vi "Voltage Update.vi"(7 "shared variable refnum in":refnum<k21>, 8 "error in (no error)":errorcluster, 9 "Amplifier Gain":dbl=1.0 min=-15.0 max=15.0, 10 "Voltage Output":dbl(slide) min=-50.0 max=50.0 scale=-45.0..45.0, 11 "Physical Channel":tag="Dev2/ao0") -> (0 "error out":errorcluster, 2 "DAQ output":dbl(slide)=-0.0 min=-3.5 max=3.5 scale=-3.5..3.5)   [LabVIEW 2016]
doc: "I. Description:\nThis example demonstrates how to output a single Voltage Update (Sample) to an Analog Output Channel.\n\nII. Instructions for Running:\n1. Select the Physical Channel to correspond to where your signal is output on the DAQ device.\n2. Enter the Minimum and Maximum Voltage Ranges\nNote: Use the Acq One Sample example to verify you are generating the correct output on the DAQ device\n\nIII. Block Diagram Steps:\n1. Create an Analog Output Voltage Channel\n2. Use the Write VI to Output 1 Sample to 1 Channel on the Data\nAcquisition Card. \n3. Call the Clear Task VI to clear the Task.\n4. Use the popup dialog box to display an error if any. \n\nIV. I/O Connections Overview:\nMake sure your signal output terminal matches the Physical Channel I/O Control. For further connection information, refer to your hardware reference manual."
uses:
  <vilib>/DAQmx/write.llb/DAQmx Write (Analog 1D DBL 1Chan NSamp).vi
  <vilib>/DAQmx/write.llb/DAQmx Write (Analog DBL 1Chan 1Samp).vi
  <vilib>/DAQmx/create/channels.llb/DAQmx Create Channel (AO-Voltage-Basic).vi
  <vilib>/DAQmx/configure/timing.llb/DAQmx Timing (Sample Clock).vi
  <vilib>/DAQmx/miscellaneous.llb/DAQmx Fill In Error Info.vi
  <resource>/objmgr/daqmx.rc
  <resource>/objmgr/ni.var.rc
panel:
  in  "Maximum Value":dbl=3.5
  in  "Minimum Value":dbl=-3.5 min=-3.5 max=0.0
  # "Waveform Settings"
  # "Channel Settings"
  # "Instructions"
  # "-This VI will set a DC output to a NI USB-4431 DSA DAQ\n-The absolute limits are +/- 3.5 V\n- The voltage will be maintained even when the VI is not running & if LabVIEW is shutdown"
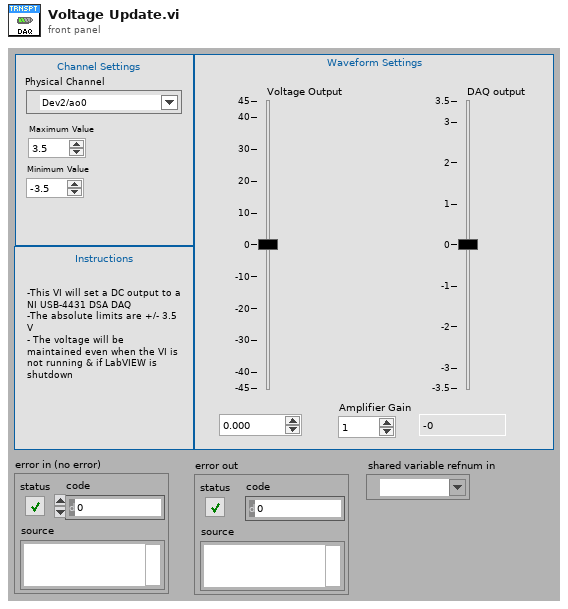
[diagram p1: front panel]
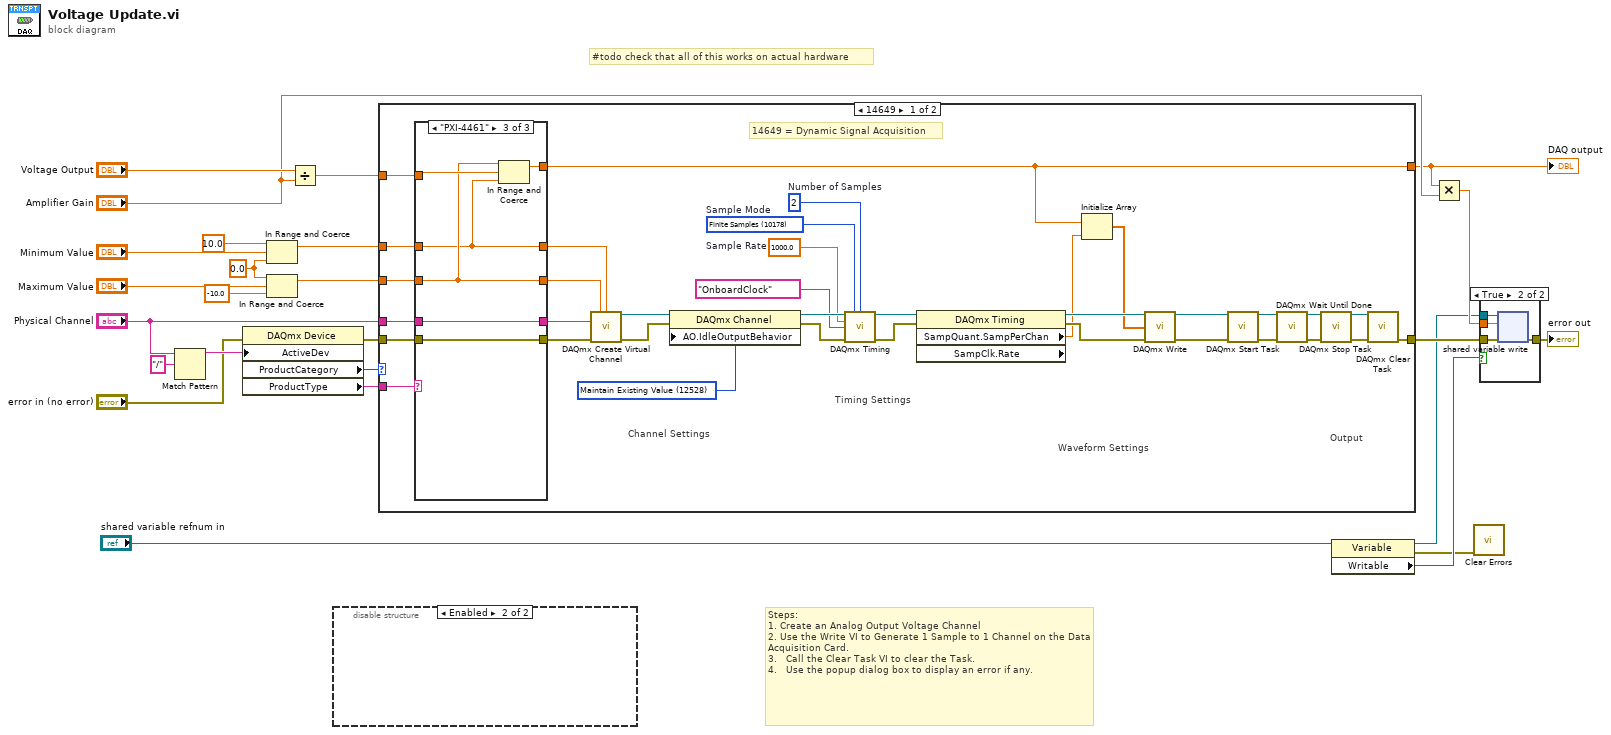
[diagram p0: block diagram]
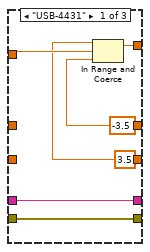
[diagram p3: hidden frame]
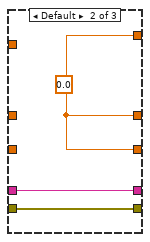
[diagram p4: hidden frame]
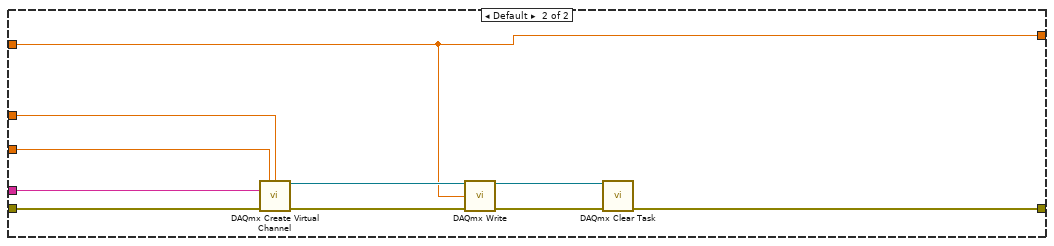
[diagram p5: hidden frame]
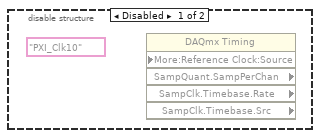
[diagram p6: hidden frame]
diagram:
  w11 = 0.0 ("upper limit")
  # "#todo check that all of this works on actual hardware"
  # "Steps: \n1. Create an Analog Output Voltage Channel\n2. Use the Write VI to Generate 1 Sample to 1 Channel on the Data Acquisition Card.  \n3.   Call the Clear Task VI to clear the Task.\n4.   Use the popup dialog box to display an error if any."
  n1 = Match Pattern(string="Physical Channel", regular expression="/") -> (before substring=w24:string)  [unwired: 1 in, 3 out]
  n2 = property class="DAQmx Device"(error in="error in (no error)", "ActiveDev"=w24) -> (error out=w23:errorcluster, "ProductCategory"=w21:i32, "ProductType"=w19:string)  [unwired: 1 in, 1 out]
  n3 = In Range and Coerce(upper limit=10.0, x="Minimum Value", lower limit=w11) -> (coerced(x)=w13:dbl)  [unwired: 1 out]
  n4 = In Range and Coerce(upper limit=w11, x="Maximum Value", lower limit=-10.0) -> (coerced(x)=w12:dbl)  [unwired: 1 out]
  n5 = Divide(x="Voltage Output", y="Amplifier Gain") -> (x/y=w20:dbl)
  n6 = disable-structure shown="Enabled" {
    frame Disabled {
      (unwired) tag "PXI_Clk10" ("RefClk.Src")
      n7 = property class="DAQmx Timing" props=["More:Reference Clock:Source", "SampQuant.SampPerChan", "SampClk.Timebase.Rate", "SampClk.Timebase.Src"]() -> ()  [unwired: 3 in, 5 out]
    }
    frame Enabled {
    }
  }
  n8 = case shown="14649" w21 {
    tunnel: [w29 w77] -> w10
    tunnel: w23 -> [w30 w81]
    tunnel: "Physical Channel" -> [w33 w80]
    tunnel: w20 -> [w34 w76]
    tunnel: w19 -> [w60 _]
    tunnel: w12 -> [w37 w79]
    tunnel: w13 -> [w35 w78]
    tunnel: [w26 w76] -> w5
    frame 14649 {
      w49 = 2  # Number of Samples
      w43 = 1000.0  # Sample Rate
      w57 = 12528 items=["Zero Volts"=12526, "High-Impedance"=12527, "Maintain Existing Value"=12528] ("AO.IdleOutputBehavior")
      w40 = 10178 items=["Finite Samples"=10178, "Continuous Samples"=10123, "Hardware Timed Single Point"=12522]  # Sample Mode
      # "Output"
      # "Waveform Settings"
      # "Timing Settings"
      # "Channel Settings"
      # "14649 = Dynamic Signal Acquisition"
      n9 = case shown="\"PXI-4461\"" w60 {
        tunnel: [w65 w69 w73] -> w38
        tunnel: w37 -> [_ _ w73]
        tunnel: [w64 w69 w72] -> w36
        tunnel: w35 -> [_ _ w72]
        tunnel: w34 -> [w66 _ w75]
        tunnel: [w63 w69 w74] -> w26
        tunnel: w33 -> [w62 w67 w70]
        tunnel: [w62 w67 w70] -> w32
        tunnel: [w61 w68 w71] -> w31
        tunnel: w30 -> [w61 w68 w71]
        frame "USB-4431" {
          w65 = 3.5 ("Maximum Value")
          w64 = -3.5 ("Minimum Value")
          n10 = In Range and Coerce(upper limit=w65, x=w66, lower limit=w64) -> (coerced(x)=w63:dbl)  [unwired: 1 out]
        }
        frame Default {
          w69 = 0.0 ("Maximum Value")
        }
        frame "PXI-4461" {
          n11 = In Range and Coerce(upper limit=w73, x=w75, lower limit=w72) -> (coerced(x)=w74:dbl)  [unwired: 1 out]
        }
      }
      n12 = call-poly <vilib>:"DAQmx Create Virtual Channel.vi"("maximum value"=w38, "minimum value"=w36, "physical channels"=w32, "error in"=w31) -> ("task out"=w41:refnum<k21>, "error out"=w55:errorcluster)  [unwired: 10 in]
      n13 = property class="DAQmx Channel"(reference=w41, error in=w55, "AO.IdleOutputBehavior"=w57) -> (reference out=w54:refnum<k21>, error out=w56:errorcluster)
      n14 = call-poly <vilib>:"DAQmx Timing.vi"("task/channels in"=w54, "sample mode"=w40, "samples per channel"=w49, "rate"=w43, "source"=tag "OnboardClock" ("Sample Clock Source"), "error in"=w56) -> ("task out"=w39:refnum<k21>, "error out"=w59:errorcluster)  [unwired: 8 in]
      n15 = property class="DAQmx Timing" props=["SampQuant.SampPerChan", "SampClk.Rate"](reference=w39, error in=w59) -> (reference out=w44:refnum<k21>, error out=w58:errorcluster, "SampQuant.SampPerChan"=w27:dbl)  [unwired: 1 out]
      n16 = Initialize Array(w26, w27) -> (w28:dbl[])
      n17 = call-poly <vilib>:"DAQmx Write.vi"("task/channels in"=w44, "data"=w28, "error in"=w58) -> ("task out"=w45:refnum<k21>, "error out"=w46:errorcluster)  [unwired: 10 in, 1 out]
      n18 = call <vilib>:"DAQmx Start Task.vi"("task/channels in"=w45, "error in"=w46) -> ("task out"=w47:refnum<k21>, "error out"=w48:errorcluster)  [unwired: 12 in]
      n19 = call <vilib>:"DAQmx Wait Until Done.vi"("task/channels in"=w47, "error in"=w48) -> ("task out"=w52:refnum<k21>, "error out"=w53:errorcluster)  [unwired: 12 in]
      n20 = call <vilib>:"DAQmx Stop Task.vi"("task/channels in"=w52, "error in"=w53) -> ("task out"=w50:refnum<k21>, "error out"=w51:errorcluster)  [unwired: 12 in]
      n21 = call <vilib>:"DAQmx Clear Task.vi"("task in"=w50, "error in"=w51) -> ("error out"=w29:errorcluster)  [unwired: 13 in]
    }
    frame Default {
      n22 = call-poly <vilib>:"DAQmx Create Virtual Channel.vi"("maximum value"=w79, "minimum value"=w78, "physical channels"=w80, "error in"=w81) -> ("task out"=w85:refnum<k21>, "error out"=w84:errorcluster)  [unwired: 10 in]
      n23 = call-poly <vilib>:"DAQmx Write.vi"("task/channels in"=w85, "data"=w76, "error in"=w84) -> ("task out"=w82:refnum<k21>, "error out"=w83:errorcluster)  [unwired: 10 in, 1 out]
      n24 = call <vilib>:"DAQmx Clear Task.vi"("task in"=w82, "error in"=w83) -> ("error out"=w77:errorcluster)  [unwired: 13 in]
    }
  }
  "DAQ output" <- w5
  n25 = property class="Variable"(reference="shared variable refnum in") -> (reference out=w2:refnum<k21>, error out=w1:errorcluster, "Writable"=w3:bool)  [unwired: 1 in]
  n26 = Multiply(x=w5, y="Amplifier Gain") -> (x*y=w6:dbl)
  n27 = call <vilib>:"Clear Errors.vi"("error in (no error)"=w1) -> ()  [unwired: 5 in, 2 out]
  n28 = case shown="True" w3 {
    tunnel: w10 -> [w86 w90]
    tunnel: [w86 w89] -> w9
    tunnel: w6 -> [_ w88]
    tunnel: w2 -> [_ w87]
    frame False {
    }
    frame True {
      n29 = shared-variable-write(w87, w90, w88) -> (w89:errorcluster)  [unwired: 1 out]
    }
  }
  "error out" <- w9
